vi "CreatPoints.vi"(3 "Wave Ticks":u32=80, 4 "Ramp Offset":dbl, 6 "Ramp Amplitude":dbl=1.0, 7 "offset":dbl caption="Triangle Offset" format="%0.2p", 8 "Triangle Amplitude":dbl=1.0, 9 "Triangle Phase":dbl=270.0, 10 "Triangle Frequency":dbl=1000.0, 11 "Signal Type":T1(ring)=enum."Triangle Wave") -> (0 "Sample Rate":dbl=500000.0 format="%#_6p", 1 "Ramp Out":i16[](array[numeric]), 2 "Triangle Out":i16[](array[numeric]))   [LabVIEW 2015]
uses:
  <vilib>/measure/NI_MABase.lvlib
panel:
  out "x+y":dbl
  out "The First":i16
  out "The Last":i16
  out "最小值":i16
  out "最大值":i16
  out "Sample Number":i32=10000
  out "波形图":i16[][](graph)
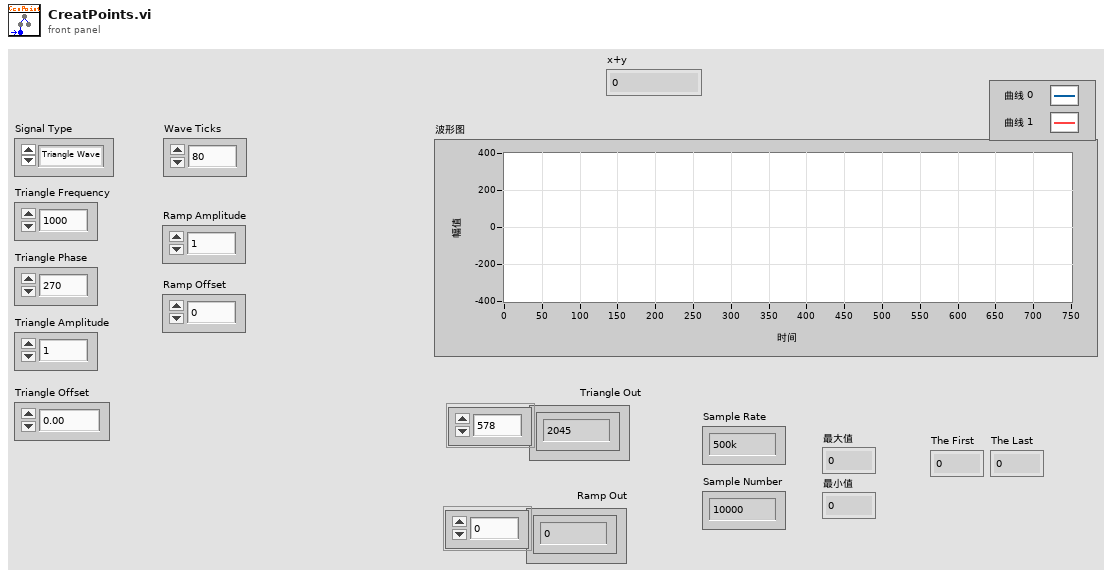
[diagram p1: front panel]
types:
  T1 = enum16{"Sine Wave", "Triangle Wave", "Square Wave", "Sawtooth Wave"}
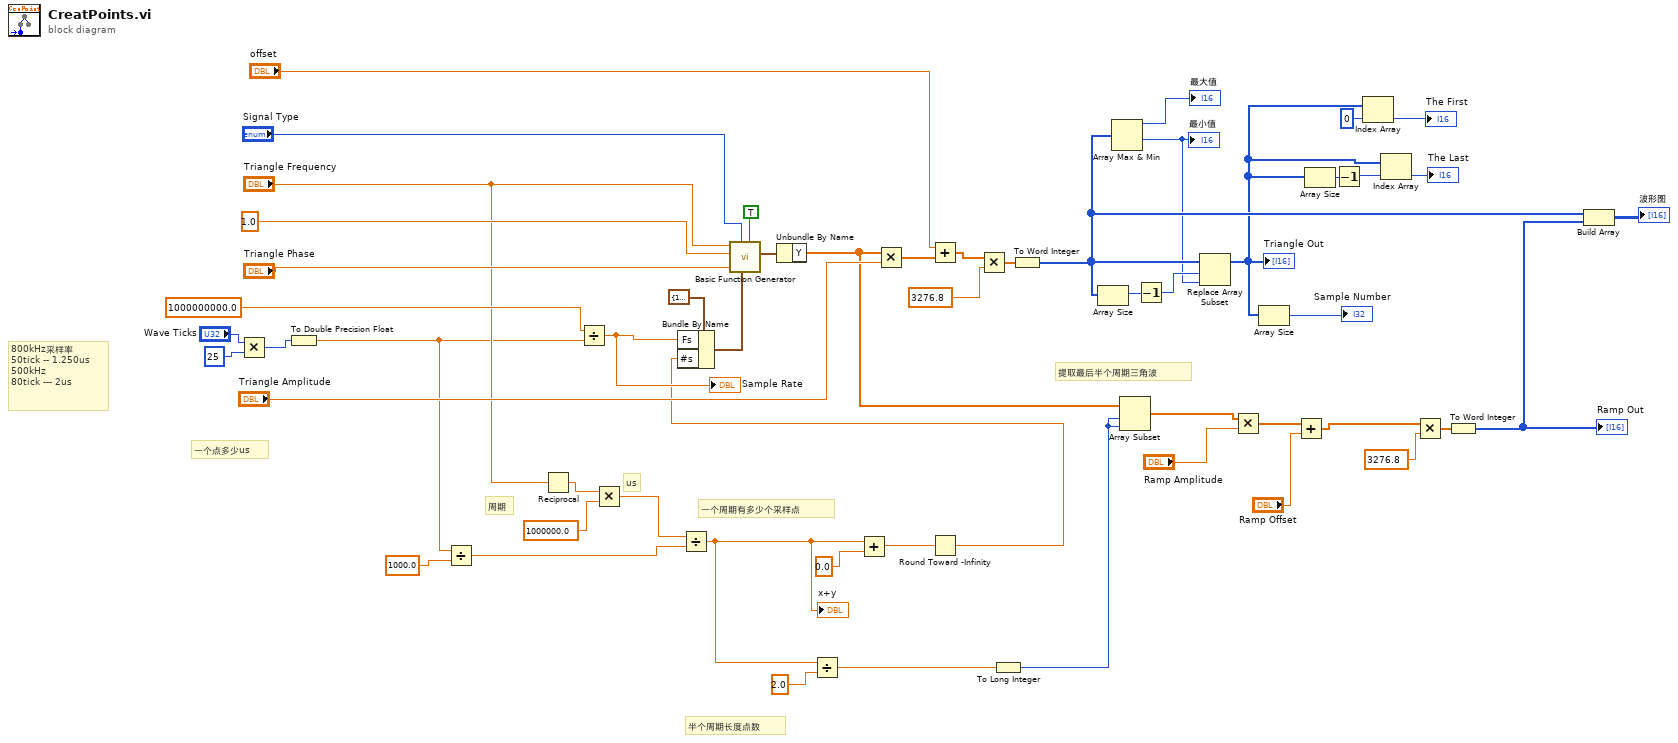
[diagram p0: block diagram]
diagram:
  # "半个周期长度点数"
  # "提取最后半个周期三角波"
  # "一个周期有多少个采样点"
  # "一个点多少us"
  # "us"
  # "周期"
  # "800kHz采样率\n50tick -- 1.250us\n500kHz\n80tick --- 2us"
  n1 = Multiply(x="Wave Ticks", y=u32 25) -> (x*y=w40:u32)
  n2 = To Double Precision Float(number=w40) -> (double precision float=w30:dbl)
  n3 = Divide(x=w30, y=1000.0) -> (x/y=w36:dbl)
  n4 = Reciprocal(x="Triangle Frequency") -> (1/x=w35:dbl)
  n5 = Divide(x=1000000000.0 ("t"), y=w30) -> (x/y=w41:dbl)
  "Sample Rate" <- w41
  n6 = Multiply(x=w35, y=1000000.0) -> (x*y=w34:dbl)
  n7 = Divide(x=w34, y=w36) -> (x/y=w3:dbl)
  "x+y" <- w3
  n8 = Divide(x=w3, y=2.0) -> (x/y=w28:dbl)
  n9 = Add(x=w3, y=0.0) -> (x+y=w2:dbl)
  n10 = Round Toward -Infinity(1:w2) -> (0:w1:dbl)
  n11 = Bundle By Name(cluster=cluster{"Fs":dbl, "#s":dbl} {"Fs"=1000.0, "#s"=1000.0} ("sampling info"), "Fs"=w41, "#s"=w1) -> (w48:cluster{"Fs":dbl, "#s":dbl})
  n12 = call <vilib>:"Basic Function Generator.vi"("reset signal"=TRUE, "sampling info"=w48, "signal type"="Signal Type", "phase"="Triangle Phase", "amplitude"=1.0, "frequency"="Triangle Frequency") -> ("signal out"=w45:waveform(dbl))  [unwired: 3 in, 2 out]
  n13 = Unbundle By Name(w45) -> ("Y"=w26:dbl[])
  n14 = Multiply(x=w26, y="Triangle Amplitude") -> (x*y=w21:dbl[])
  n15 = Add(x="offset", y=w21) -> (x+y=w22:dbl[])
  n16 = Multiply(x=w22, y=3276.8 ("amplitude")) -> (x*y=w53:dbl[])
  n17 = To Long Integer(number=w28) -> (32bit integer=w27:i32)
  n18 = To Word Integer(number=w53) -> (16bit integer=w9:i16[])
  n19 = Array Size(array=w9) -> (size(s)=w8:i32)
  n20 = Array Max & Min(array=w9) -> (max value=→"最大值":i16, min value=w6:i16)  [unwired: 2 out]
  "最小值" <- w6
  n21 = Array Subset(array=w26, index=w27, length=w27) -> (w18:dbl[])
  n22 = Decrement(x=w8) -> (x-1=w7:i32)
  n23 = Replace Array Subset(array=w9, new element=w6, index=w7) -> (w5:i16[])
  "Triangle Out" <- w5
  n24 = Multiply(x=w18, y="Ramp Amplitude") -> (x*y=w17:dbl[])
  n25 = Array Size(array=w5) -> (size(s)=→"Sample Number":i32)
  n26 = Add(x=w17, y="Ramp Offset") -> (x+y=w16:dbl[])
  n27 = Array Size(array=w5) -> (size(s)=w15:i32)
  n28 = Decrement(x=w15) -> (x-1=w11:i32)
  n29 = Index Array(array=w5, index=0 ("索引")) -> (element=→"The First":i16)
  n30 = Index Array(array=w5, index=w11) -> (element=→"The Last":i16)
  n31 = Multiply(x=w16, y=3276.8 ("amplitude")) -> (x*y=w32:dbl[])
  n32 = To Word Integer(number=w32) -> (16bit integer=w19:i16[])
  "Ramp Out" <- w19
  n33 = Build Array(w9, w19) -> (→"波形图":i16[][])
